vi "1.7.vi"() -> ()   [LabVIEW 2017]
panel:
  out "String":string
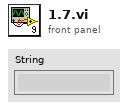
[diagram p1: front panel]
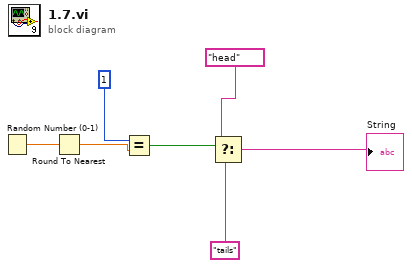
[diagram p0: block diagram]
diagram:
  n1 = Random Number (0-1)() -> (number: 0 to 1=w7:dbl)
  n2 = Round To Nearest(number=w7) -> (nearest integer value=w3:dbl)
  n3 = Equal?(x=1, y=w3) -> (x = y?=w1:bool)
  n4 = Select(t="head", s=w1, f="tails") -> (s? t:f=→"String":string)
